vi "ExSetSerialRegClns.vi"() -> ()   [LabVIEW 2010]
uses:
  Open-Close Hardware/CamHandle.vi
panel:
  out "error out":errorcluster
  in  "error in (no error)":errorcluster
  in  "skip serial  reg clean":dbl=1.0 format="%.2f"
  # "ExSetSerialRegClns.vi : This vi sets up the \nserial register cleans. Note: not all cameras\nsupport this function."
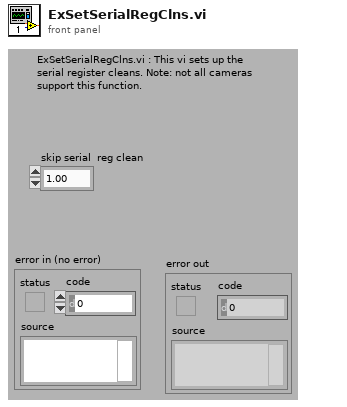
[diagram p1: front panel]
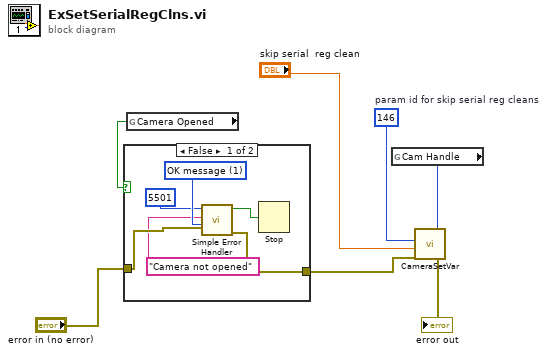
[diagram p0: block diagram]
diagram:
  w1 = 146  # param id for skip serial reg cleans
  n1 = global read "CamHandle.vi" "Camera Opened"() -> (w7:bool)
  n2 = case shown="False" w7 {
    tunnel: "error in (no error)" -> [w12 w14]
    tunnel: [w11 w14] -> w3
    frame False {
      w13 = u16 1 items=["no dialog", "OK message", "continue or stop message"] ("type of dialog (OK msg:1)")
      n3 = call <vilib>:"Simple Error Handler.vi"("error code (no error:0)"=5501, "error source (\" \")"="Camera not opened", "type of dialog (OK msg:1)"=w13, "error in (no error)"=w12) -> ("error?"=w9:bool, "error out"=w11:errorcluster)  [unwired: 1 in, 3 out]
      n4 = Stop(stop? (T)=w9) -> ()
    }
    frame True {
    }
  }
  n5 = global read "CamHandle.vi" "Cam Handle"() -> (w4:u32)
  n6 = call <userlib>:"CameraSetVar.vi"("error in"=w3, "Value"="skip serial  reg clean", "Parameter ID"=w1, "Camera Handle"=w4) -> ("error out"=→"error out":errorcluster)  [unwired: 1 out]
